vi "reconnect.vi"(8 "error in (no error)":errorcluster, 11 "TCPClient in":refnum<class "TCPClient.lvclass">) -> (0 "error out":errorcluster, 3 "TCPClient out":refnum<class "TCPClient.lvclass">)   [LabVIEW 2016, in "TCPClient.lvclass"]
uses:
  TCPClient.lvclass
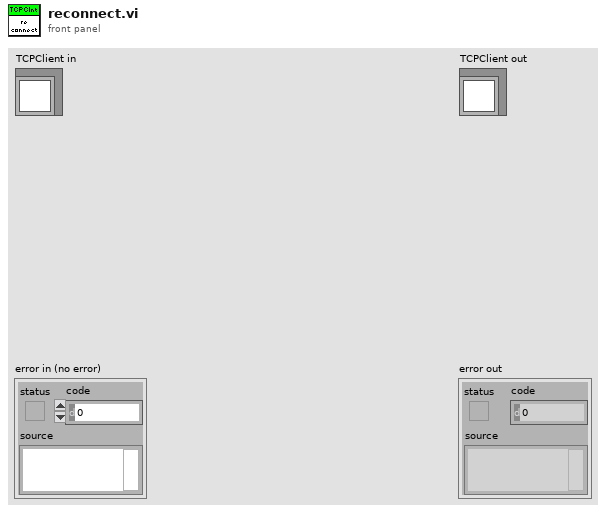
[diagram p1: front panel]
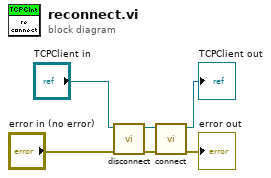
[diagram p0: block diagram]
diagram:
  n1 = call-dynamic "disconnect.vi"("error in (no error)"="error in (no error)", "TCPClient in"="TCPClient in") -> ("error out"=w1:errorcluster, "TCPClient out"=w2:refnum<class "TCPClient.lvclass">)  [unwired: 7 in, 1 out]
  n2 = call-dynamic "connect.vi"("error in (no error)"=w1, "TCPClient in"=w2) -> ("error out"=→"error out":errorcluster, "TCPClient out"=→"TCPClient out":refnum<class "TCPClient.lvclass">)  [unwired: 8 in]
